vi "Destroy.vi"(0 "reference in":refnum<class "Electric ECU.lvclass">, 11 "Error In":errorcluster) -> (4 "reference out":refnum<class "Electric ECU.lvclass">, 15 "Error Out":errorcluster)   [LabVIEW 2024, in "Electric ECU.lvclass"]
uses:
  Electric ECU.lvclass/Electric ECU.ctl
  Electric ECU.lvclass
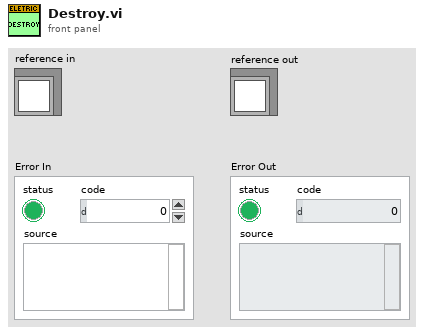
[diagram p1: front panel]
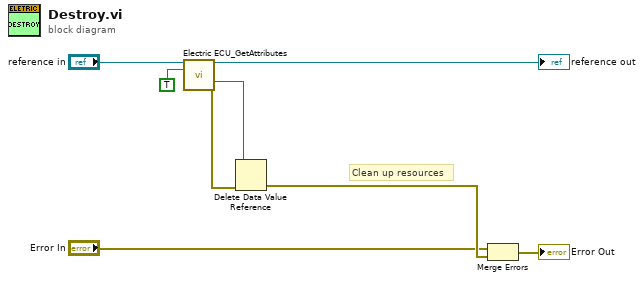
[diagram p0: block diagram]
diagram:
  # "Clean up resources"
  n1 = call "Electric ECU_GetAttributes.vi"("reference in"="reference in", "OnlyGetDvrReference(False)"=TRUE) -> ("reference out"=→"reference out":refnum<class "Electric ECU.lvclass">, "DataRef"=w4:refnum<data-value>, "Error Out"=w5:errorcluster)  [unwired: 10 in, 1 out]
  n2 = Delete Data Value Reference(data value reference=w4, error in=w5) -> (error out=w3:errorcluster)  [unwired: 1 out]
  n3 = Merge Errors("Error In", w3) -> (→"Error Out":errorcluster)
